vi "readInXMLNative.vi"(8 "error in (no error)":errorcluster, 10 "scriptEventXML":refnum<k20>, 11 "Delay in":refnum<class "Delay.lvclass">) -> (0 "error out":errorcluster, 3 "Delay out":refnum<class "Delay.lvclass">)   [LabVIEW 2009, in "Tools.lvlib" / "Scripting.lvlib" / "Delay.lvclass"]
uses:
  Delay.lvclass
  <vilib>/xml/Close Reference(Node).vi
  ScriptEvent.lvclass
  <vilib>/xml/NI_XML.lvlib
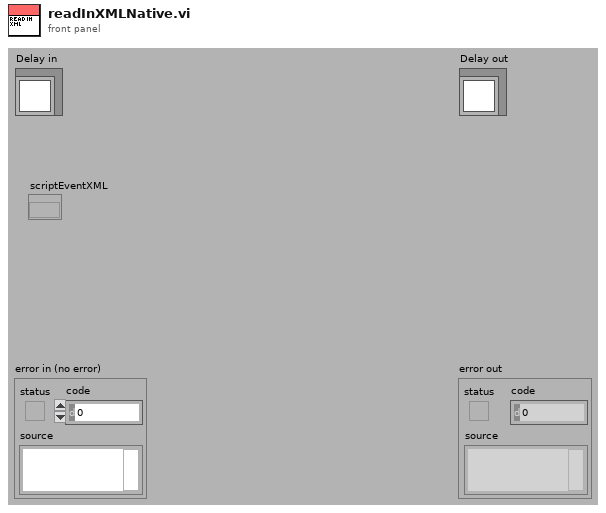
[diagram p1: front panel]
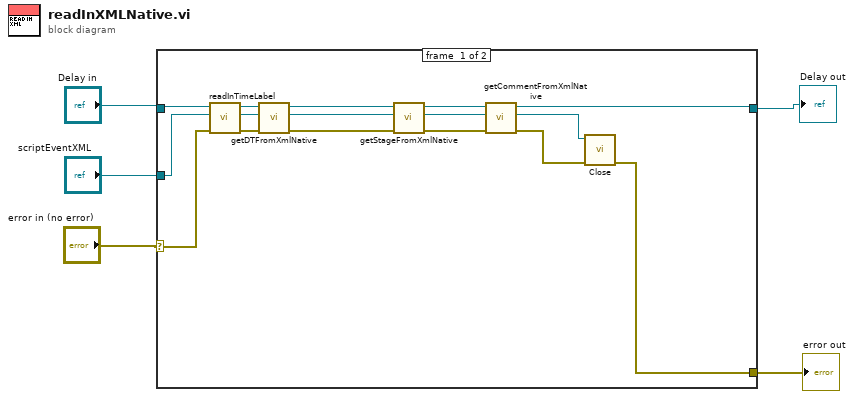
[diagram p0: block diagram]
diagram:
  n1 = case shown="No Error" "error in (no error)" {
    selector: "error in (no error)" -> [w12 w23]
    tunnel: [w18 w23] -> w1
    tunnel: [w11 w22] -> w2
    tunnel: "Delay in" -> [w14 w22]
    tunnel: "scriptEventXML" -> [w13 _]
    frame #0 {
      n2 = call "readInTimeLabel.vi"("error in (no error)"=w12, "eventXML"=w13, "Delay in"=w14) -> ("error out"=w15:errorcluster, "eventXML out"=w16:refnum<k20>, "Delay out"=w17:refnum<class "Delay.lvclass">)  [unwired: 6 in]
      n3 = call "getDTFromXmlNative.vi"("error in (no error)"=w15, "eventXML"=w16, "ScriptEvent in"=w17) -> ("error out"=w8:errorcluster, "eventXML out"=w6:refnum<k20>, "ScriptEvent out"=w7:refnum<class "Delay.lvclass">)  [unwired: 6 in]
      n4 = call "getStageFromXmlNative.vi"("error in (no error)"=w8, "eventXML"=w6, "ScriptEvent in"=w7) -> ("error out"=w20:errorcluster, "eventXML out"=w19:refnum<k20>, "ScriptEvent out"=w21:refnum<class "Delay.lvclass">)  [unwired: 6 in]
      n5 = call "getCommentFromXmlNative.vi"("error in (no error)"=w20, "eventXML"=w19, "ScriptEvent in"=w21) -> ("error out"=w9:errorcluster, "eventXML out"=w10:refnum<k20>, "ScriptEvent out"=w11:refnum<class "Delay.lvclass">)  [unwired: 6 in]
      n6 = call-poly <vilib>:"Close.vi"("error in (no error)"=w9, "node"=w10) -> ("error out"=w18:errorcluster)  [unwired: 7 in]
    }
    frame #1 {
    }
  }
  "error out" <- w1
  "Delay out" <- w2
